vi "Scan_Hopping with IT at Surface.vi"() -> ()   [LabVIEW 2023]
uses:
  Sub_Vi/TypeDefs/Settings.ctl
  Sub_Vi/TypeDefs/ChangeOnFly.ctl
  Sub_Vi/TypeDefs/Display.ctl
  Settings.vi
panel:
  in  "ABSOLUTE Distance To Retrack at line end/ um":dbl=1.0
  in  "V2":dbl
  in  "Feedback Type":T1(ring)
  in  "IT Time2 / s":dbl
  in  "IT Time1 / s":dbl
  in  "Retract After Scan":bool=TRUE
  in  "IT Time / s":dbl
  in  "Display Cluster":T2
  in  "ChangeonFly":T3
  in  "SettingsCluster":T4={"Sample Rate (us)"=1, "Samples Per Data Point (int, power of 2)"=1000, "DistanceToBulk (um)"=-1.0, "HoldTimeScaler"=40000, "SaveData"=TRUE, "DistanceToBulk (um) 2"=-1.0, "DistanceToBulk (um) 3"=-1.0}
  in  "Greater Than":bool=TRUE
  in  "V1":dbl
  in  "Approach Rate Hopping (um/s)":dbl=1.0
  in  "Retrack Rate (um/s)":dbl=1.0
  in  "HoppingDistance":dbl=1.0
  in  "Z End":dbl=38.0
  in  "ABSOLUTE Distance To Retrack / um":dbl=1.0
  in  "Upper dZ limit":i32=8
  in  "Feedback Threshold\nAbsolute value":dbl=1e-13
  in  "P":fxp<+/-,32,1> format="%.32g"
  in  "X Center":dbl=150.0 min=0.0 max=300.0
  in  "Y Center":dbl=150.0 min=0.0 max=300.0
  in  "Y Width":dbl=10.0
  in  "X Width":dbl=10.0
  in  "Lateral Scan Rate (um/s)":dbl=1.0
  in  "V":dbl=1.0
  in  "Z Start height":dbl
  in  "Start scan Button":bool
  in  "Stop":bool
  in  "Pause":bool
  out "Y end":dbl
  out "X end":dbl
  out "X start":dbl
  out "Y start":dbl
  in  "Tab Control 4":enum32{"AC Approach", "AC Approach 2"}(tab)
  out "Waveform Graph 2":dbl[](graph)
  out "Waveform Graph":dbl[](graph)
  out "XY Graph":cluster{"Y":dbl[], "Y":dbl[]}[](graph)
  out "Waveform Graph 4":dbl[](graph)
  out "Waveform Graph 3":dbl[](graph)
  # "Scaning protocols"
  # "At Surface"
  # "V2"
  # "V2 (Retract)"
  # "IT Time2 / s"
  # "V1"
  # "Feedback  Settings"
  # "IT Time1 / s"
  # "V (Approach)"
  # "V"
  # "V (Move to the next point)"
  # "IT Time / s"
  # "Initial Approach  Settings"
  # "Scan  Settings"
  # "Max of IT Times should be EITHER below 32 seconds OR above 32 seconds"
  # "This value is ADDED to the piezo position"
  # "Define Scan area \nAbout centre"
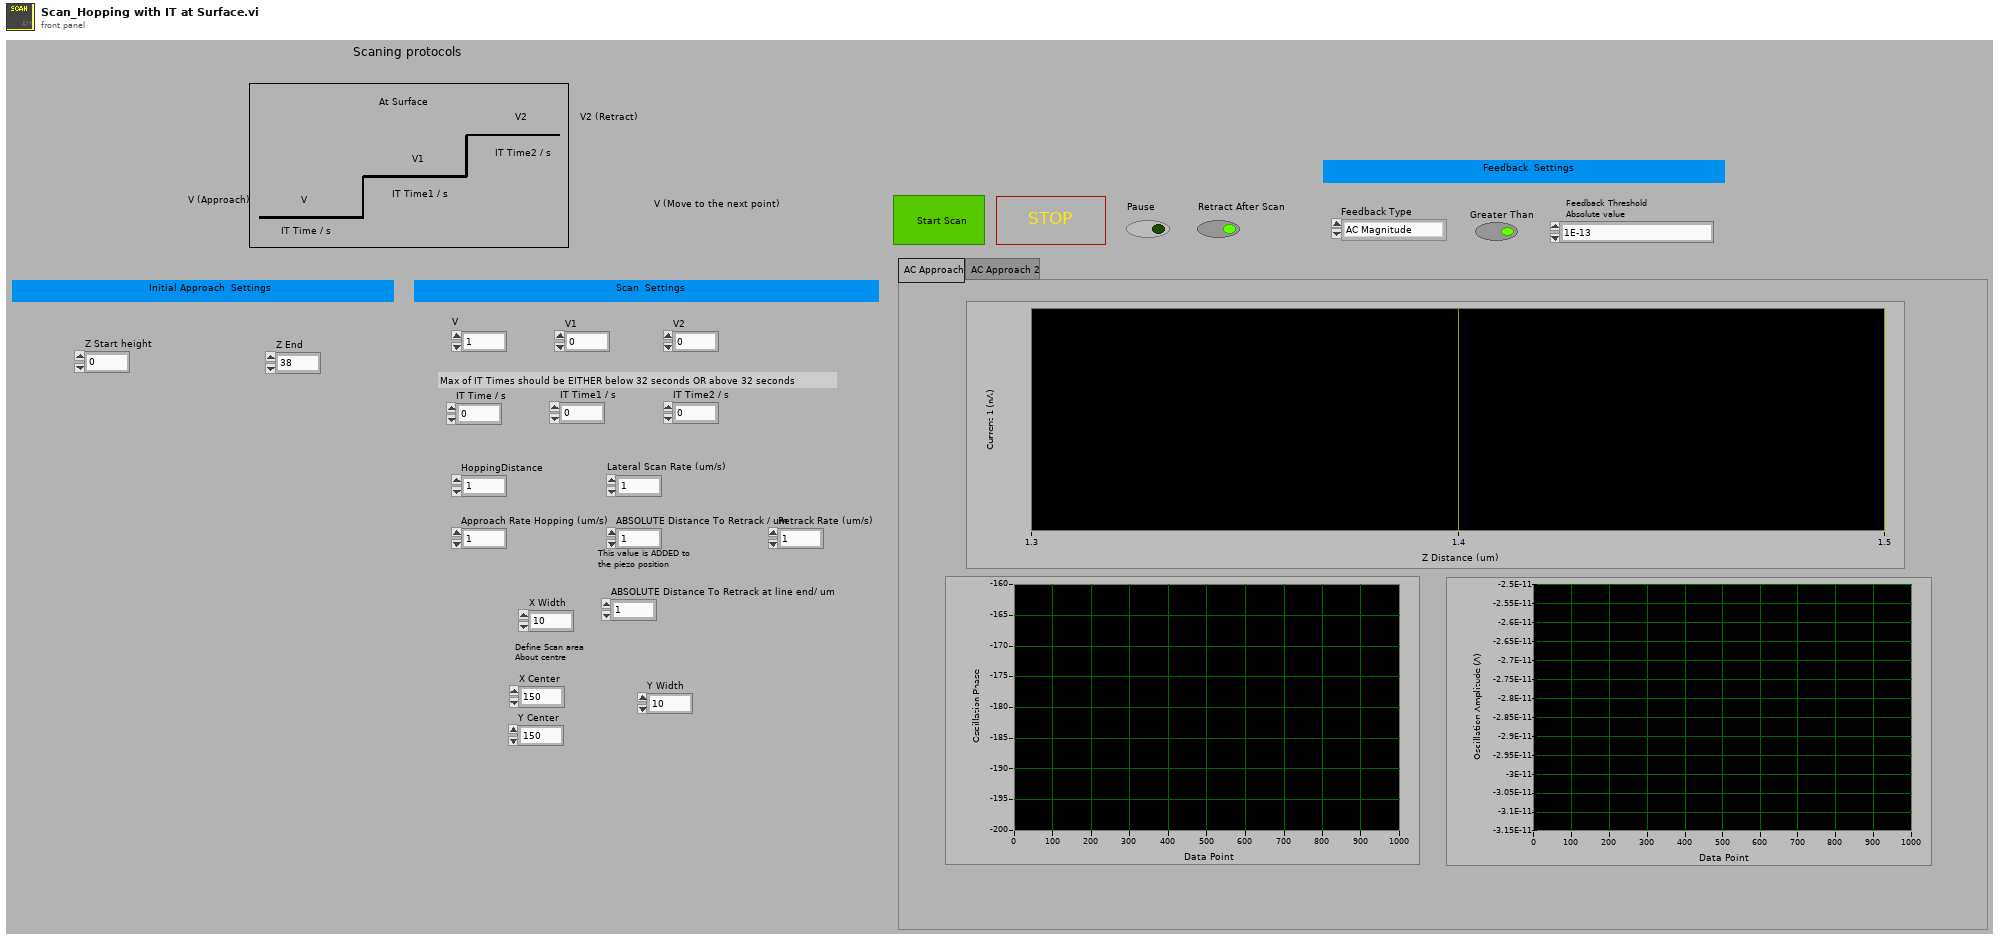
[diagram p1: front panel]
types:
  T1 = enum16{"AC Magnitude", "Current 1", "Current 2", "Phase"}
  T2 = typedef "Display.ctl" = cluster{"X":refnum<vi>, "Y":refnum<vi>, "Z":refnum<vi>, "Amp":refnum<vi>, "Phase":refnum<vi>, "t vs Z":refnum<vi>, "t vs C1":refnum<vi>, "t vs C2":refnum<vi>, "t vs C3":refnum<vi>, "t vs Amp":refnum<vi>, "t vs Phase":refnum<vi>, "t vs X":refnum<vi>, "t vs Y":refnum<vi>, "Z vs C1":refnum<vi>, "Z vs C2":refnum<vi>, "Z vs C3":refnum<vi>, "V vs C1":refnum<vi>, "V vs C2":refnum<vi>, "V vs C3":refnum<vi>, "X/Y/Z F":refnum<vi>, "X/Y/Z R":refnum<vi>, "X/Y/C1 F":refnum<vi>, "X/Y/C1 R":refnum<vi>, "X/Y/C2 F":refnum<vi>, "X/Y/C2 R":refnum<vi>, "X/Y/C3 F":refnum<vi>, "X/Y/C3 R":refnum<vi>, "NumberOfLines":u16, "um Per Pixel":dbl, "um Per Line":dbl, "X Center":dbl, "Hop X/Y/Z":refnum<vi>, "Hop X/Y/C1":refnum<vi>, "Hop X/Y/C2":refnum<vi>, "Hop X/Y/C3":refnum<vi>, "X Width":dbl, "Y Width":dbl, "Hopping Distance":dbl, "V2 vs C1":refnum<vi>, "V vs Phase":refnum<vi>, "Y Center":dbl, "Number of Pixels":dbl, "V2 vs C2":refnum<vi>, "V2 vs C3":refnum<vi>, "V vs y":refnum<vi>, "V2 vs y":refnum<vi>, "Z vs Amp":refnum<vi>, "Z vs Phase":refnum<vi>}
  T3 = typedef "ChangeOnFly.ctl" = cluster{"Stop (boolean)":refnum<vi>, "Pause (boolean)":refnum<vi>, "EndCurrentLine (boolean)":refnum<vi>, "max movement per update step (Interger, nm)":refnum<vi>, "P (float, arb)":refnum<vi>, "Feedback set point (double, Amps)":refnum<vi>, "Voltage (double, V)":refnum<vi>, "Feedback set point 2 (double, Amps)":refnum<vi>, "Stop on Greater Than 2? (boolean)":refnum<vi>, "Stop on Greater Than? (boolean)":refnum<vi>, "Voltage 2 (double, V)":refnum<vi>, "Feedback Type (enum)":refnum<vi>, "Feedback Type 2 (enum)":refnum<vi>}
  T4 = typedef "Settings.ctl" = cluster{"Sample Rate (us)":u32, "Samples Per Data Point (int, power of 2)":i16, "DistanceToBulk (um)":dbl, "HoldTimeScaler":u64, "SaveData":bool, "DistanceToBulk (um) 2":dbl, "DistanceToBulk (um) 3":dbl}
  T5 = cluster{"Scan Rate (um/s)":dbl, "X Start":dbl, "X End":dbl, "Y Start":dbl, "Y End":dbl, " Z Start":dbl, "HoppingDistance":dbl, "V":dbl, "Z End":dbl, "Approach Rate Hopping (um/s)":dbl, "Retrack Rate (um/s)":dbl, "V 1":dbl, "HoldTime IT/s":dbl, "HoldTime Bulk Pre IT/s 2":dbl, "HoldTime Bulk IT Post/s":dbl, "V2":dbl, "HoldTime Bulk IT Post/s 4":dbl}
  T6 = typedef "WayPointCluster.ctl" = cluster{"X (um)":dbl[], "Y (um)":dbl[], "Z (um)":dbl[], "V (V)":dbl[], "X Velocity (um s-1)":dbl[], "Y Velocity (um s-1)":dbl[], "Z Velocity (um s-1)":dbl[], "V Velocity (V s-1)":dbl[], "FeedBack Type (enum)":u16[], "Move X (boolean)":bool[], "Move Y (boolean)":bool[], "Move Z (boolean)":bool[], "Move V (boolean)":bool[], "Jump V (boolean)":bool[], "Hold (boolean)":bool[], "Hold Time":u32[], "V2 (V)":dbl[], "Move V2":bool[], "V2 Velocity (V s-1)":dbl[], "Jump V2 (boolean)":bool[], "Update z Position delta (ms)":i16[], "Hold Feedback1":bool[], "Move Z PicoMotor":bool[], " Z PicoMotor Direction":bool[], "DIO0":bool[]}
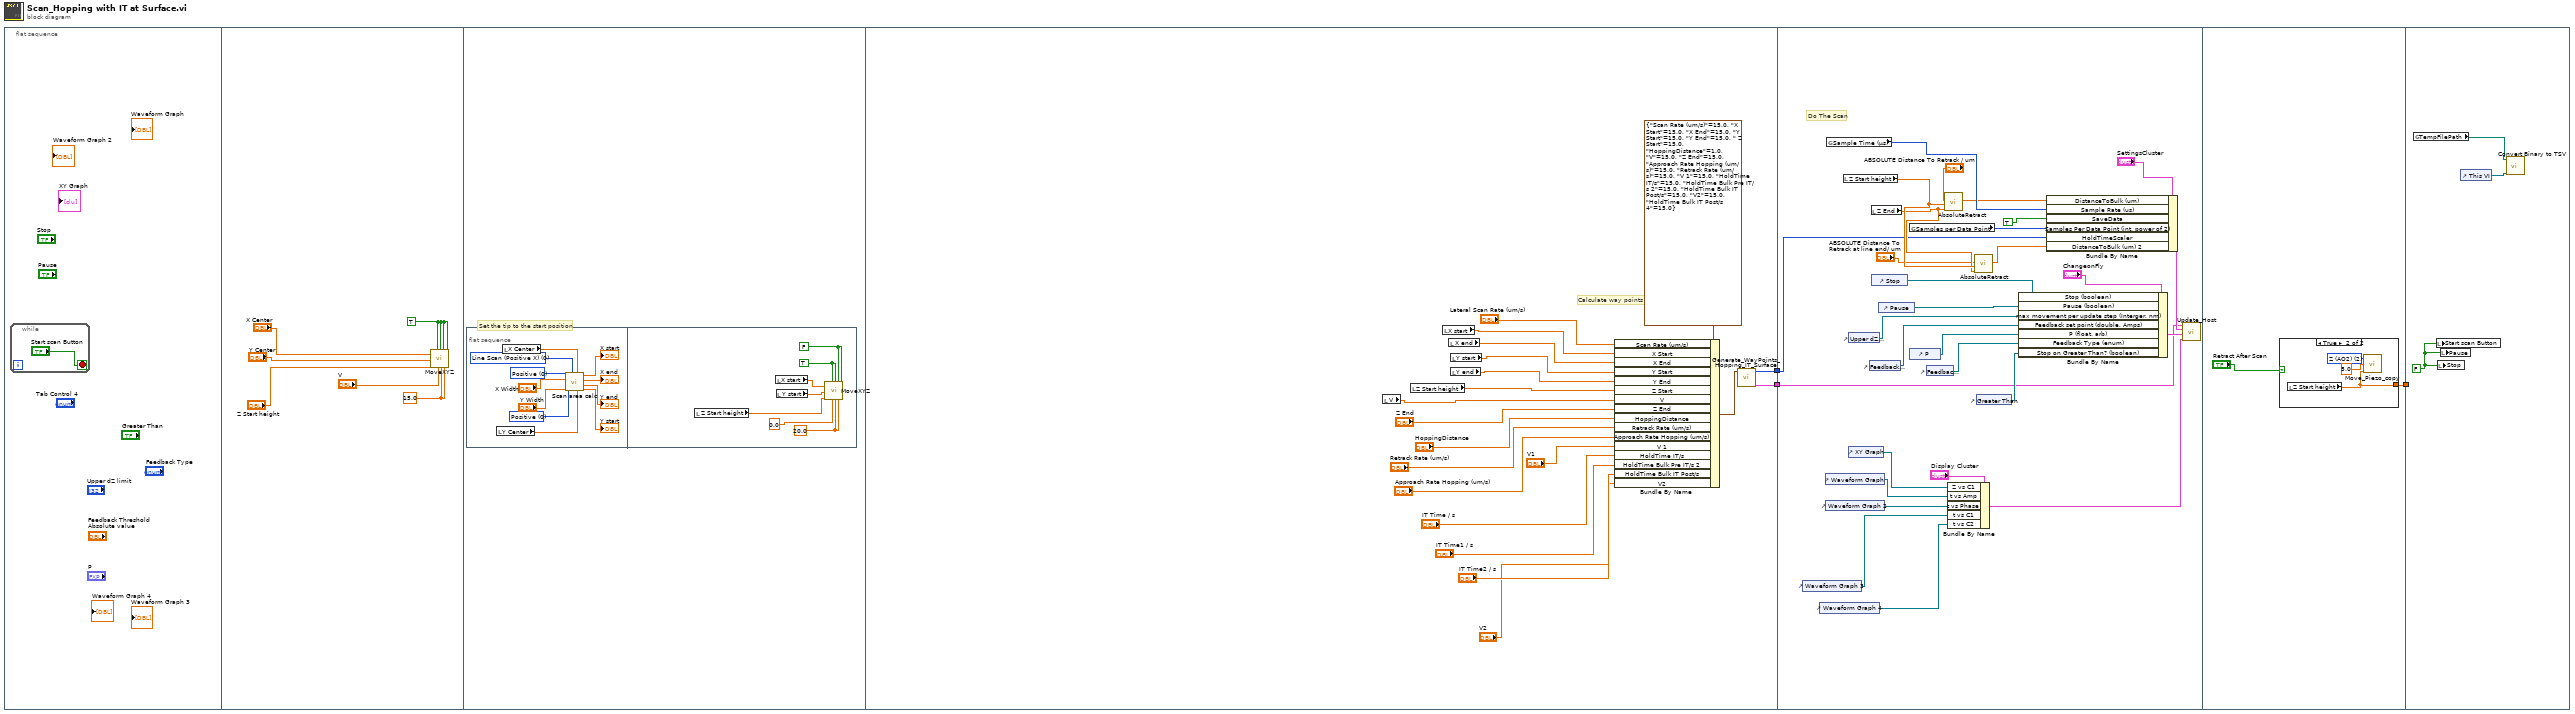
[diagram p0: block diagram]
diagram:
  n1 = flat-sequence {
    tunnel: [w32] -> w2
    tunnel: [w30] -> w1
    tunnel: w2 -> [w57]
    tunnel: w1 -> [w49]
    tunnel: [w78] -> w3
    tunnel: w3 -> [_]
    frame #0 {
      n2 = while {
        stop <- "Start scan Button" stop-if-true
      }
    }
    frame #1 {
      w5 = TRUE ("Set X")
      w10 = 15.0 ("Scan Rate (V/s) X and Y")
      n3 = call "MoveXYZ.vi"("X final height"="X Center", "Y final height"="Y Center", "Z final height"="Z Start height", "Set X"=w5, "V final"="V", "Set Y"=w5, "Scan Rate (um/s)"=w10, "Set Z"=w5, "Scan Rate (V/s) 2"=w10, "Set Voltage"=w5) -> ()  [unwired: 10 in]
    }
    frame #2 {
      # "Set the tip to the start position"
      n4 = flat-sequence {
        frame #0 {
          w11 = u16 0 items=["Positive", "Negative"] ("Major Axis Direction")
          w12 = u16 0 items=["Positive", "Negative"] ("Minor Axis Direction")
          w13 = u16 0 items=["Line Scan (Positive X)", "Line Scan (Negative X)", "Line Scan (Positive Y)", "Line Scan (Negative Y)"] ("Scan Type")
          n5 = local read "Y Center"() -> (w14:dbl)
          n6 = local read "X Center"() -> (w15:dbl)
          n7 = call "Scan area calc.vi"("Y Width"="Y Width", "Major Axis Direction"=w11, "X Width"="X Width", "Minor Axis Direction"=w12, "Scan Type"=w13, "Y Center"=w14, "X Center"=w15) -> ("Y start"=→"Y start":dbl, "Y end"=→"Y end":dbl, "X end"=→"X end":dbl, "X start"=→"X start":dbl)
        }
        frame #1 {
          w22 = FALSE ("Set Z")
          w23 = TRUE ("Set X")
          w24 = 20.0 ("Scan Rate (V/s)")
          n8 = local read "Z Start height"() -> (w28:dbl)
          n9 = local read "X start"() -> (w26:dbl)
          n10 = local read "Y start"() -> (w27:dbl)
          n11 = call "MoveXYZ.vi"("X final height"=w26, "Y final height"=w27, "Z final height"=w28, "Set X"=w23, "V final"=0.0 ("Scan Rate (V/s) X and Y"), "Set Y"=w23, "Scan Rate (um/s)"=w24, "Set Z"=w22, "Scan Rate (V/s) 2"=w24, "Set Voltage"=w22) -> ()  [unwired: 10 in]
        }
      }
    }
    frame #3 {
      # "Calculate way points for the Scan"
      n12 = local read "V"() -> (w36:dbl)
      n13 = local read "Z Start height"() -> (w43:dbl)
      n14 = local read "X start"() -> (w47:dbl)
      n15 = local read "X end"() -> (w46:dbl)
      n16 = local read "Y start"() -> (w45:dbl)
      n17 = local read "Y end"() -> (w44:dbl)
      n18 = Bundle By Name(cluster=T5 {"Scan Rate (um/s)"=15.0, "X Start"=15.0, "X End"=15.0, "Y Start"=15.0, "Y End"=15.0, " Z Start"=15.0, "HoppingDistance"=1.0, "V"=15.0, "Z End"=15.0, "Approach Rate Hopping (um/s)"=15.0, "Retrack Rate (um/s)"=15.0, "V 1"=15.0, "HoldTime IT/s"=15.0, "HoldTime Bulk Pre IT/s 2"=15.0, "HoldTime Bulk IT Post/s"=15.0, "V2"=15.0, "HoldTime Bulk IT Post/s 4"=15.0} ("Input Cluster"), "Scan Rate (um/s)"="Lateral Scan Rate (um/s)", "X Start"=w47, "X End"=w46, "Y Start"=w45, "Y End"=w44, "Z Start"=w43, "V"=w36, "Z End"="Z End", "HoppingDistance"="HoppingDistance", "Retrack Rate (um/s)"="Retrack Rate (um/s)", "Approach Rate Hopping (um/s)"="Approach Rate Hopping (um/s)", "V 1"="V1", "HoldTime IT/s"="IT Time / s", "HoldTime Bulk Pre IT/s 2"="IT Time1 / s", "HoldTime Bulk IT Post/s"="IT Time2 / s", "V2"="V2") -> (w29:T5)
      n19 = call "Generate_WayPoints_Hopping_IT_Surface.vi"("Input Cluster"=w29) -> ("output cluster"=w32:T6, "WaitTimeScaler"=w30:u64)  [unwired: 9 in]
    }
    frame #4 {
      # "Do The Scan"
      n20 = control-ref of="Waveform Graph 3"() -> (w65:refnum<vi>)
      n21 = control-ref of="Waveform Graph 4"() -> (w64:refnum<vi>)
      n22 = control-ref of="Waveform Graph"() -> (w76:refnum<vi>)
      n23 = control-ref of="Waveform Graph 2"() -> (w75:refnum<vi>)
      n24 = global read "Settings.vi" "Sample Time (µs)"() -> (w60:u32)
      n25 = local read "Z Start height"() -> (w54:dbl)
      n26 = control-ref of="Upper dZ limit"() -> (w71:refnum<vi>)
      n27 = control-ref of="XY Graph"() -> (w77:refnum<vi>)
      n28 = control-ref of="Feedback Threshold\nAbsolute value"() -> (w69:refnum<vi>)
      n29 = local read "Z End"() -> (w53:dbl)
      n30 = control-ref of="Stop"() -> (w66:refnum<vi>)
      n31 = control-ref of="Pause"() -> (w67:refnum<vi>)
      n32 = control-ref of="P"() -> (w70:refnum<vi>)
      n33 = global read "Settings.vi" "Samples per Data Point"() -> (w59:u16)
      n34 = control-ref of="Feedback Type"() -> (w50:refnum<vi>)
      n35 = call "AbsoluteRetract.vi"("Z End"=w53, "Z Start height"=w54, "Distance To Retract / um"="ABSOLUTE Distance To Retrack / um") -> ("Distance To Retract / um 2"=w56:dbl)  [unwired: 8 in]
      n36 = Bundle By Name(cluster="Display Cluster", "Z vs C1"=w77, "t vs Amp"=w76, "t vs Phase"=w75, "t vs C1"=w65, "t vs C2"=w64) -> (w74:T2)
      n37 = call "AbsoluteRetract.vi"("Z End"=w53, "Z Start height"=w54, "Distance To Retract / um"="ABSOLUTE Distance To Retrack at line end/ um") -> ("Distance To Retract / um 2"=w51:dbl)  [unwired: 8 in]
      n38 = control-ref of="Greater Than"() -> (w58:refnum<vi>)
      n39 = Bundle By Name(cluster="ChangeonFly", "Stop (boolean)"=w66, "Pause (boolean)"=w67, "max movement per update step (Interger, nm)"=w71, "Feedback set point (double, Amps)"=w69, "P (float, arb)"=w70, "Feedback Type (enum)"=w50, "Stop on Greater Than? (boolean)"=w58) -> (w72:T3)
      n40 = Bundle By Name(cluster="SettingsCluster", "DistanceToBulk (um)"=w56, "Sample Rate (us)"=w60, "SaveData"=TRUE ("Save Data"), "Samples Per Data Point (int, power of 2)"=w59, "HoldTimeScaler"=w49, "DistanceToBulk (um) 2"=w51) -> (w73:T4)
      n41 = call "Update_Host.vi"("Display Cluster"=w74, "ChangeonFly"=w72, "SettingsCluster"=w73, "WayPointCluster"=w57) -> ()  [unwired: 6 in]
    }
    frame #5 {
      n42 = case shown="True" "Retract After Scan" {
        tunnel: [_ w80] -> w78
        frame False {
        }
        frame True {
          w82 = u16 2 items=["X (AO0)", "Y (AO1)", "Z (AO2)", "V (AO3)"] ("Channel")
          n43 = local read "Z Start height"() -> (w80:dbl)
          n44 = call "Move_Piezo_copy.vi"("Piezo"=w82, "Movement Speed (µm/s)"=5.0 ("Scan Rate (um/s)"), "Position (µm) (or V)"=w80) -> ()  [unwired: 13 in]
        }
      }
    }
    frame #6 {
      w85 = FALSE ("Stop")
      n45 = global read "Settings.vi" "TempFilePath"() -> (w83:path)
      n46 = local write "Start scan Button"(w85) -> ()
      n47 = local write "Stop"(w85) -> ()
      n48 = local write "Pause"(w85) -> ()
      n49 = control-ref of="This VI"() -> (w84:refnum<vi>)
      n50 = call "Convert Binary to TSV.vi"("This VI"=w84, "TDMS DataFile Name"=w83) -> ()  [unwired: 10 in]
    }
  }
